vi "gfitsio-read-image-subset-i16-3d.vi"(4 "lpixel (-1,-1,-1: rest)":cluster{"X":i32, "Y":i32, "Z":i32}={"X"=-1, "Y"=-1, "Z"=-1}, 6 "fpixel (1,1,1)":cluster{"X":i32, "Y":i32, "Z":i32}={"X"=1, "Y"=1, "Z"=1}, 7 "inc (1,1,1)":cluster{"X":i32, "Y":i32, "Z":i32}={"X"=1, "Y"=1, "Z"=1}, 8 "error in (no error)":errorcluster, 9 "nulval (0: don't check)":i16, 11 "gfits refnum":T1) -> (0 "error out":errorcluster, 1 "anynul":bool, 2 "data":i16[][][](array[numeric]), 3 "dup gfits refnum":T1)   [LabVIEW 2015]
doc: "Read a rectangular subimage (or the whole image) from the FITS data array. <B>fpixel</B> and <B>lpixel</B> give the coordinates of the first (lower left corner) and last (upper right corner) pixels to be read from the FITS image. Undefined FITS array elements will be set equal to <B>nullval</B> unless <B>nulval</B> is zero in which case no checks for undefined pixels will be performed."
uses:
  gfitsio.lvlib
  cfitsio-datatypes.ctl
  gfitsio_32Bit/gfitsio.dll
  gfitsio_32Bit/gfitsio-refnum.ctl
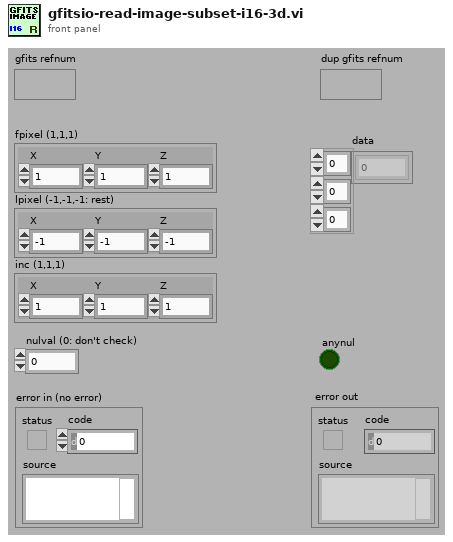
[diagram p1: front panel]
types:
  T1 = typedef "gfitsio-refnum.ctl" = refnum<k1>
  T2 = typedef "gfitsio.lvlib/gfitsio-refnum.ctl" = refnum<k1>
  T3 = typedef "gfitsio.lvlib/cfitsio-datatypes.ctl" = i32
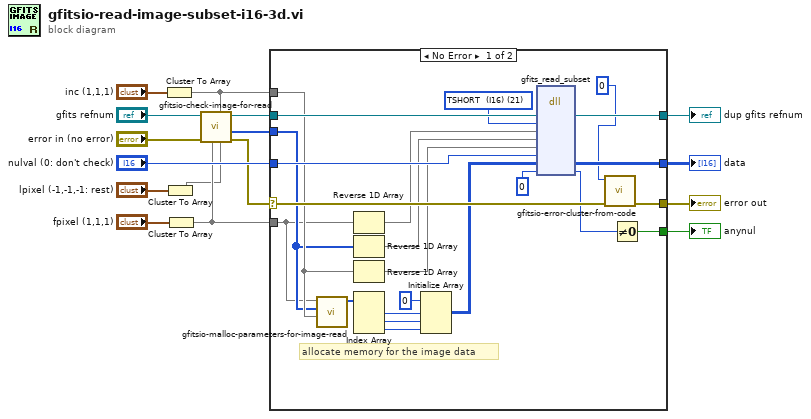
[diagram p0: block diagram]
diagram:
  n1 = Cluster To Array(cluster="inc (1,1,1)") -> (array=w1:i32[])
  n2 = Cluster To Array(cluster="lpixel (-1,-1,-1: rest)") -> (array=w2:i32[])
  n3 = Cluster To Array(cluster="fpixel (1,1,1)") -> (array=w3:i32[])
  n4 = call "gfitsio-check-image-for-read.vi"("inc out"=w2, "npixels out"=w1, "inc"=w3, "error in (no error)"="error in (no error)", "gfits refnum"="gfits refnum") -> ("error out"=w5:errorcluster, "lpixel out"=w4:i32[], "dup gfits refnum"=w10:T2)  [unwired: 3 in, 1 out]
  n5 = case shown="No Error" w5 {
    selector: w5 -> [w35 w40]
    tunnel: [w39 w40] -> w15
    tunnel: w10 -> [w37 w41]
    tunnel: [w36 w41] -> w16
    tunnel: "nulval (0: don't check)" -> [w34 _]
    tunnel: [w32 _] -> w13
    tunnel: [w31 _] -> w12
    tunnel: w3 -> [w24 _]
    tunnel: w4 -> [w25 _]
    tunnel: w1 -> [w26 _]
    frame No Error {
      w30 = T3 21 items=["TBIT"=1, "TBYTE  (U8)"=11, "TSBYTE  (I8)"=12, "TLOGICAL"=14, "TSTRING"=16, "TUSHORT  (U16)"=20, "TSHORT  (I16)"=21, "TUINT"=31, "TULONG  (U32)"=40, "TLONG  (I32)"=41, "TFLOAT  (SGL)"=42, "TLONGLONG  (I64)"=81, "TDOUBLE  (DBL)"=82, "TCOMPLEX  (CSG)"=83, "TDOUBLECOMPLEX  (CDB)"=163] ("cfitsio datatype")
      # "allocate memory for the image data"
      n6 = call "gfitsio-malloc-parameters-for-image-read.vi"("inc"=w26, "lpixel"=w25, "fpixel"=w24) -> ("image dimensions"=w21:i32[])  [unwired: 8 in]
      n7 = Reverse 1D Array(array=w24) -> (reversed array=w27:i32[])
      n8 = Reverse 1D Array(array=w25) -> (reversed array=w28:i32[])
      n9 = Reverse 1D Array(array=w26) -> (reversed array=w29:i32[])
      n10 = Index Array(array=w21) -> (element #1=w20:i32, element #2=w19:i32, element #3=w18:i32)  [unwired: 3 in]
      n11 = Initialize Array(i16 0 ("element"), w20, w19, w18) -> (w22:i16[][][])
      n12 = dll-call lib="C:/GSCS 2.0/GSCS/Systems/SIcamera_Control/Quick_Look/gfitsio_32Bit/gfitsio.dll" fn="gfits_read_subset"("handle"=w37, "datatype"=w30, "fpixel"=w27, "lpixel"=w28, "inc"=w29, "nulval"=w34, "array"=w22, "anynul"=0) -> ("handle"=w36:T2, "array"=w31:i16[][][], "anynul"=w33:i32)  [unwired: 9 in, 2 out]
      n13 = call "gfitsio-error-cluster-from-code.vi"("error in (no error)"=w35, "error code"=0) -> ("error out"=w39:errorcluster)  [unwired: 9 in]
      n14 = Not Equal To 0?(x=w33) -> (x != 0?=w32:bool)
    }
    frame Error {
    }
  }
  "dup gfits refnum" <- w16
  "error out" <- w15
  "anynul" <- w13
  "data" <- w12
